vi "FPGA Main.vi"() -> ()   [LabVIEW 2015]
doc: "This FPGA Main VI contains a control loop running in parallel with an RT watchdog loop.\n- The Control Loop performs control calculations on four input channels in parallel, and outputs the results to four output channels.\n- The RT Watchdog Loop checks for a periodic 'pet' from the RT Main VI to ensure communications between RT and FPGA are maintained."
uses:
  <vilib>/LabVIEW Targets/FPGA/cRIO/shared/nicrio_ModuleControls/nicrio_cRIO-9234_DataRatesRing2.ctl
  <vilib>/rvi/Emulation/niFpgaGetClockAttributes.vi
  <vilib>/rvi/Emulation/niFpgaSctlEmulationGetInTimedLoop.vi
  <vilib>/rvi/Emulation/niFpgaEmulationReportErrorSimple.vi
  <vilib>/rvi/Emulation/niFpgaProcessEmulError.vi
  <vilib>/rvi/eio/common/nirviEmuTemplatePropertySet_errors.vi
  <vilib>/rvi/eio/common/nirviEmuTemplateMethod_errors.vi
  <vilib>/rvi/interface/RandomDataEmulation/niFpgaRandomDataHandleErrors.vi
  <vilib>/rvi/Emulation/niFpgaCriticalErrorInLSC.vi
  <vilib>/eio/EIOPropertyNode/EIOPropertyNode.xnode
  <vilib>/eio/EIONode/EIONode.xnode
  <vilib>/rvi/DataTransferAndStorage/Container/XNode/niFpgaContainer.xnode
  <vilib>/rvi/interface/RandomDataEmulation/nirviRandomDataFpgaReadWriteTemplate.vi
  <vilib>/rvi/eio/common/nirviEmuTemplatePropertyGet_errors.vi
  <vilib>/rvi/eio/common/nirviEmuTemplatePropertyGet_noerrors.vi
  <vilib>/rvi/eio/common/nirviEmuTemplatePropertySet_noerrors.vi
panel:
  in  "Data Rate":T1=1 items=["51.200 kS/s (NI 9234)"=1, "25.600 kS/s (NI 9234)"=2, "17.067 kS/s (NI 9234)"=3, "12.800 kS/s (NI 9234)"=4, "10.240 kS/s (NI 9234)"=5, "8.533 kS/s (NI 9234)"=6, "7.314 kS/s (NI 9234)"=7, "6.400 kS/s (NI 9234)"=8, "5.689 kS/s (NI 9234)"=9, "5.120 kS/s (NI 9234)"=10, "4.654 kS/s (NI 9234)"=11, "4.267 kS/s (NI 9234)"=12, "3.938 kS/s (NI 9234)"=13, "3.657 kS/s (NI 9234)"=14, "3.413 kS/s (NI 9234)"=15, "3.200 kS/s (NI 9234)"=16, "3.012 kS/s (NI 9234)"=17, "2.845 kS/s (NI 9234)"=18, "2.695 kS/s (NI 9234)"=19, "2.560 kS/s (NI 9234)"=20, "2.438 kS/s (NI 9234)"=21, "2.328 kS/s (NI 9234)"=22, "2.226 kS/s (NI 9234)"=23, "2.133 kS/s (NI 9234)"=24, "2.048 kS/s (NI 9234)"=25, "1.969 kS/s (NI 9234)"=26, "1.896 kS/s (NI 9234)"=27, "1.829 kS/s (NI 9234)"=28, "1.765 kS/s (NI 9234)"=29, "1.707 kS/s (NI 9234)"=30, "1.652 kS/s (NI 9234)"=31]
  out "FPGA Error":errorcluster
  out "Finished":bool
  in  "Stop":bool
  out "Module Underflow":bool
  out "DMA FIFO Full":bool
  out "Different Channel Count":bool
  out "Actual Loop Period (ticks)":u32
  out "First Read":bool
  in  "Number of Channels":i32=4
  in  "Channel Scale Array":fxp<+,24,12>[](array[numeric])=[0.0, 0.0, 0.0, 0.0]
  # "General Settings"
  # "Monitoring Values"
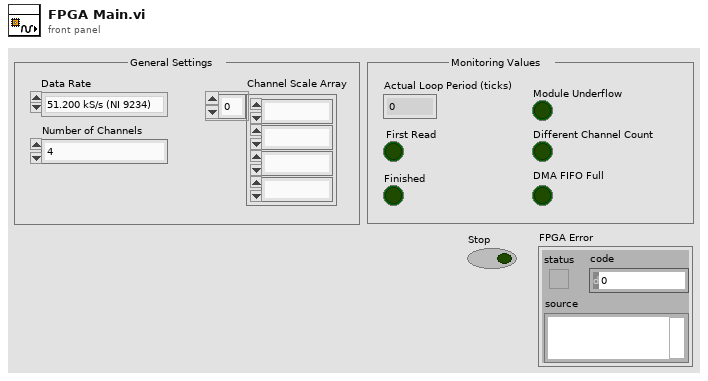
[diagram p1: front panel]
types:
  T1 = typedef "nicrio_cRIO-9234_DataRatesRing2.ctl" = u8
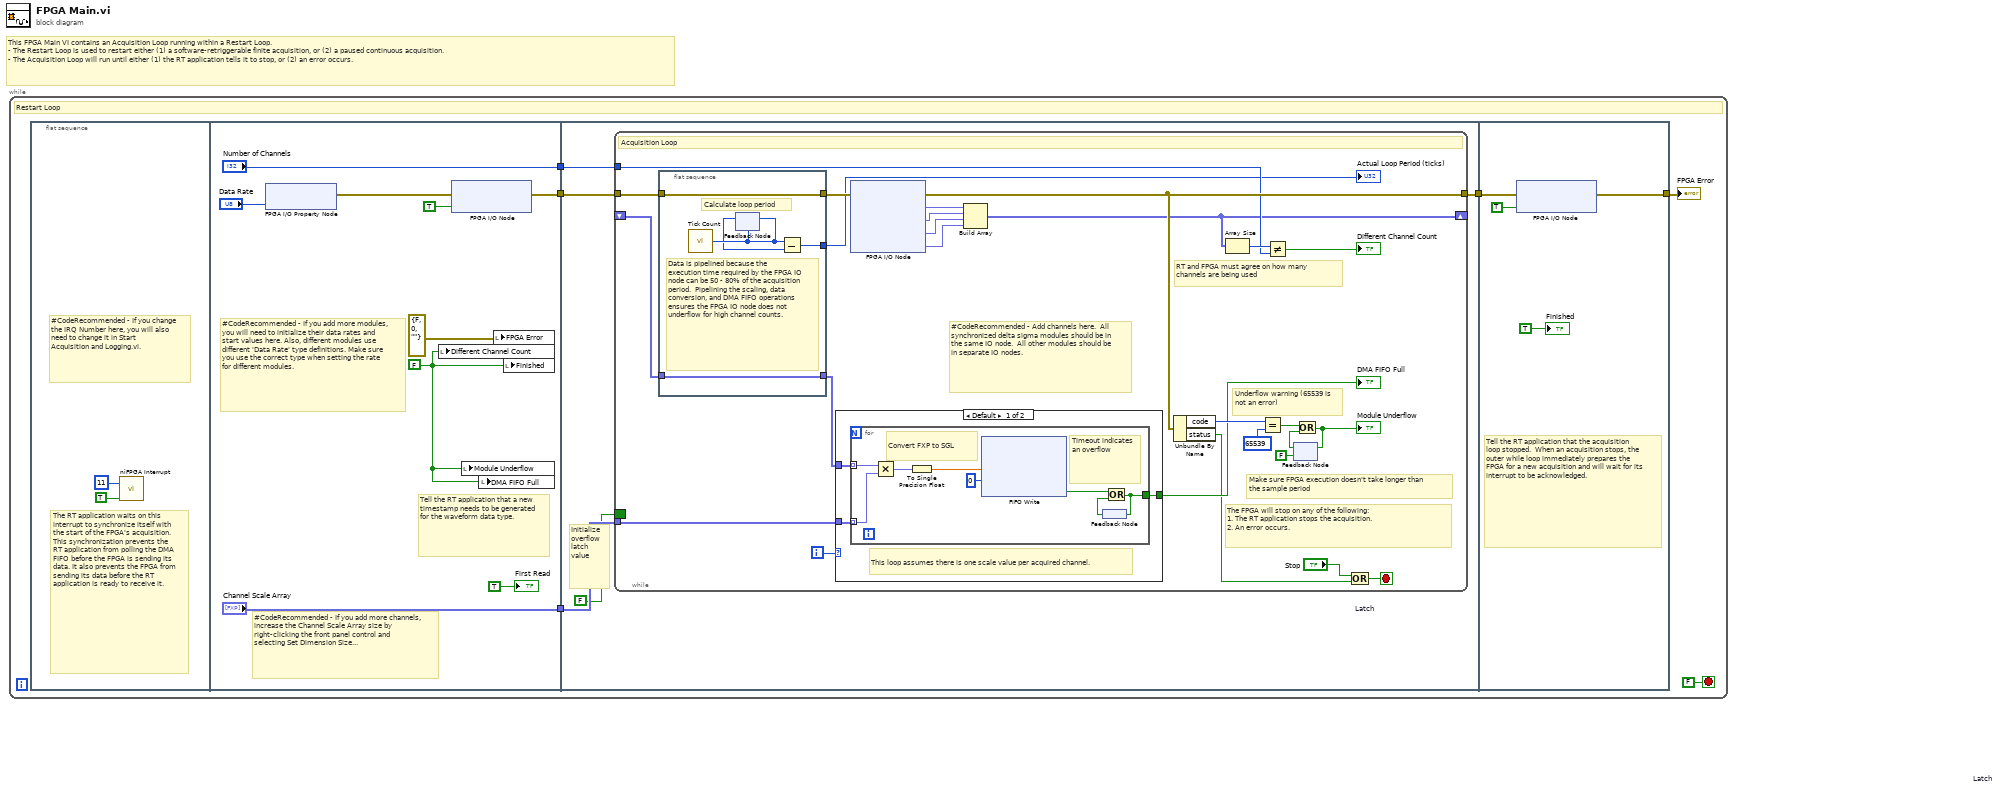
[diagram p0: block diagram]
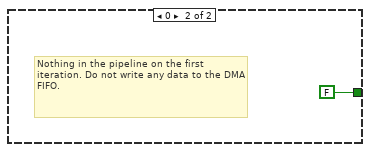
[diagram p2: hidden frame]
diagram:
  # "This FPGA Main VI contains an Acquisition Loop running within a Restart Loop.\n- The Restart Loop is used to restart either (1) a software-retriggerable finite acquisition, or (2) a paused continuous acquisition.\n- The Acquisition Loop will run until either (1) the RT application tells it to stop, or (2) an error occurs."
  n1 = while {
    stop <- FALSE stop-if-true
    # "Restart Loop"
    n2 = flat-sequence {
      tunnel: [w17] -> w5
      tunnel: ["Channel Scale Array"] -> w4
      tunnel: ["Number of Channels"] -> w3
      tunnel: w5 -> [w21]
      tunnel: w4 -> [w20]
      tunnel: w3 -> [w22]
      tunnel: [w19] -> w2
      tunnel: w2 -> [w67]
      tunnel: [w66] -> w1
      frame #0 {
        # "#CodeRecommended - If you change the IRQ Number here, you will also need to change it in Start Acquisition and Logging.vi."
        # "The RT application waits on this interrupt to synchronize itself with the start of the FPGA's acquisition.  This synchronization prevents the RT application from polling the DMA FIFO before the FPGA is sending its data. It also prevents the FPGA from sending its data before the RT application is ready to receive it."
        n3 = call <vilib>:"niFPGA Interrupt.vi"("Wait Until Cleared (F)"=TRUE ("Wait Until Cleared"), "IRQ Number (0)"=u8 11 ("IRQ Number")) -> ()  [unwired: 1 in]
      }
      frame #1 {
        w14 = FALSE ("Module Underflow")
        # "Tell the RT application that a new timestamp needs to be generated for the waveform data type."
        # "#CodeRecommended - If you add more channels, increase the Channel Scale Array size by right-clicking the front panel control and selecting Set Dimension Size..."
        # "#CodeRecommended - If you add more modules, you will need to initialize their data rates and start values here. Also, different modules use different 'Data Rate' type definitions. Make sure you use the correct type when setting the rate for different modules."
        n4 = xnode "FPGA I/O Property Node"("Data Rate"="Data Rate") -> ("error out"=w9:errorcluster)  [unwired: 2 in, 1 out]
        n5 = local write "Different Channel Count"(w14) -> ()
        n6 = xnode "FPGA I/O Node"("error in"=w9, "Mod1/Start"=TRUE) -> ("error out"=w17:errorcluster)  [unwired: 1 in, 1 out]
        n7 = local write "Module Underflow"(w14) -> ()
        n8 = local write "DMA FIFO Full"(w14) -> ()
        n9 = local write "FPGA Error"(errorcluster {"status"=FALSE, "code"=0, "source"=""} ("FPGA Error")) -> ()
        n10 = local write "Finished"(w14) -> ()
        "First Read" <- TRUE ("First Read")
      }
      frame #2 {
        # "Initialize overflow latch value"
        n11 = while {
          tunnel: w21 -> [w40]
          tunnel: [w45] -> w19
          shift-right: [w30] -> _
          shift-left: _ -> [w32]
          tunnel: w22 -> [w42]
          tunnel: w20 -> [w34]
          border: FALSE ("Overflow\nLatch") -> [_]
          i -> [w23]
          stop <- w48 stop-if-true
          # "Underflow warning (65539 is not an error)"
          # "The FPGA will stop on any of the following:\n1. The RT application stops the acquisition.\n2. An error occurs."
          # "#CodeRecommended - Add channels here.  All synchronized delta sigma modules should be in the same IO node.  All other modules should be in separate IO nodes."
          # "RT and FPGA must agree on how many channels are being used"
          # "Make sure FPGA execution doesn't take longer than the sample period"
          # "Acquisition Loop"
          n12 = flat-sequence {
            tunnel: [w65] -> w39
            tunnel: w40 -> [w65]
            tunnel: [w62] -> w38
            tunnel: w32 -> [w61]
            tunnel: [w61] -> w33
            frame #0 {
              # "Data is pipelined because the execution time required by the FPGA IO node can be 50 - 80% of the acquisition period.  Pipelining the scaling, data conversion, and DMA FIFO operations ensures the FPGA IO node does not underflow for high channel counts."
              # "Calculate loop period"
              n13 = call "Tick Count"() -> ("Tick Count(Ticks)"=w64:u32)
              n14 = feedback-in #1(w64) -> ()
              n15 = feedback #1(w64) -> (w63:u32)
              n16 = Subtract(x=w64, y=w63) -> (x-y=w62:u32)
            }
          }
          n17 = case shown="Default" w23 {
            tunnel: [w51 FALSE] -> w44
            tunnel: w34 -> [w50 _]
            tunnel: w33 -> [w49 _]
            frame Default {
              # "This loop assumes there is one scale value per acquired channel."
              n18 = for {
                tunnel: [w57] -> w51
                tunnel: w49 -> [w55] mode=indexing
                tunnel: w50 -> [w54] mode=indexing
                # "Timeout indicates an overflow"
                # "Convert FXP to SGL"
                n19 = Multiply(x=w55, y=w54) -> (x*y=w53:fxp<+/-,48,16>)
                n20 = To Single Precision Float(number=w53) -> (single precision float=w52:sgl)
                n21 = xnode ("FIFO Write")("Element"=w52, "Timeout"=0) -> ("Timed Out?"=w59:bool)  [unwired: 1 in, 1 out]
                n22 = feedback #2 "Latch"() -> (w58:bool)
                n23 = Or(x=w59, y=w58) -> (x .or. y?=w57:bool)
                n24 = feedback-in #2(w57) -> ()
              }
            }
            frame 0 {
              # "Nothing in the pipeline on the first iteration. Do not write any data to the DMA FIFO."
            }
          }
          "DMA FIFO Full" <- w44
          n25 = xnode "FPGA I/O Node"("error in"=w39) -> ("error out"=w45:errorcluster, "Mod1/AI0"=w37:fxp<+/-,24,4>, "Mod1/AI1"=w31:fxp<+/-,24,4>, "Mod1/AI2"=w36:fxp<+/-,24,4>, "Mod1/AI3"=w35:fxp<+/-,24,4>)  [unwired: 4 in, 4 out]
          n26 = Build Array(w37, w31, w36, w35) -> (w30:fxp<+/-,24,4>[])
          n27 = Unbundle By Name(w45) -> ("code"=w46:i32, "status"=w25:bool)
          n28 = Array Size(array=w30) -> (size(s)=w43:i32)
          n29 = Equal?(x=w46, y=65539) -> (x = y?=w27:bool)
          n30 = Not Equal?(x=w43, y=w42) -> (x != y?=→"Different Channel Count":bool)
          n31 = feedback #3 "Latch"(FALSE) -> (w29:bool)
          n32 = Or(x=w27, y=w29) -> (x .or. y?=w26:bool)
          "Module Underflow" <- w26
          n33 = feedback-in #3(w26) -> ()
          n34 = Compound Arithmetic op=OR("Stop", w25) -> (w48:bool)
          "Actual Loop Period (ticks)" <- w38
        }
      }
      frame #3 {
        # "Tell the RT application that the acquisition loop stopped.  When an acquisition stops, the outer while loop immediately prepares the FPGA for a new acquisition and will wait for its interrupt to be acknowledged."
        n35 = xnode "FPGA I/O Node"("error in"=w67, "Mod1/Stop"=TRUE) -> ("error out"=w66:errorcluster)  [unwired: 1 in, 1 out]
        "Finished" <- TRUE ("Finished")
      }
    }
    "FPGA Error" <- w1
  }
